vi "FeedbackNodes Test.vi"() -> ()   [LabVIEW 2014]
panel:
  out "Array 2":i32[](array[numeric])
  out "Array":i32[][](array[numeric])
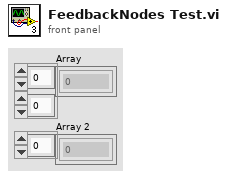
[diagram p1: front panel]
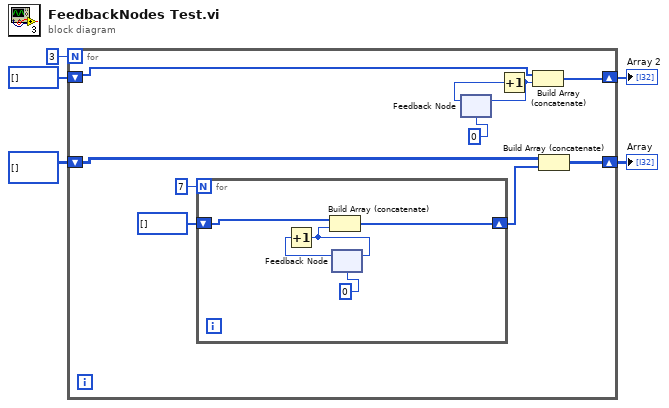
[diagram p0: block diagram]
diagram:
  n1 = for {
    N: 3 -> [_]
    shift-right: [w12] -> w3
    shift-left: i32[][] [] -> [w11]
    shift-right: [w9] -> w1
    shift-left: i32[] [] -> [w7]
    n2 = for {
      N: 7 -> [_]
      shift-right: [w20] -> w13
      shift-left: i32[] [] -> [w19]
      n3 = feedback #1(0) -> (w17:i32)
      n4 = Increment(x=w17) -> (x+1=w16:i32)
      n5 = Build Array (concatenate)(w19, w16) -> (w20:i32[])
      n6 = feedback-in #1(w16) -> ()
    }
    n7 = feedback #2(0) -> (w8:i32)
    n8 = Increment(x=w8) -> (x+1=w6:i32)
    n9 = feedback-in #2(w6) -> ()
    n10 = Build Array (concatenate)(w7, w6) -> (w9:i32[])
    n11 = Build Array (concatenate)(w11, w13) -> (w12:i32[][])
  }
  "Array" <- w3
  "Array 2" <- w1
